vi "get_curr_position.vi"(8 "error in (no error)":errorcluster, 11 "XPS in":refnum<class "XPS.lvclass">) -> (0 "error out":errorcluster, 2 "readback position":dbl[](array[numeric]), 3 "XPS out":refnum<class "XPS.lvclass">)   [LabVIEW 2019, in "XPS.lvlib" / "XPS.lvclass"]
uses:
  XPS.lvclass
  XPS.lvclass/XPS.ctl
  Newport.XPS.CommandInterface
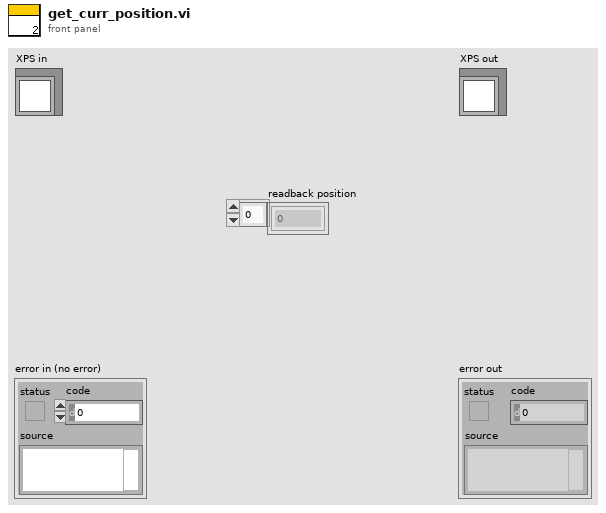
[diagram p1: front panel]
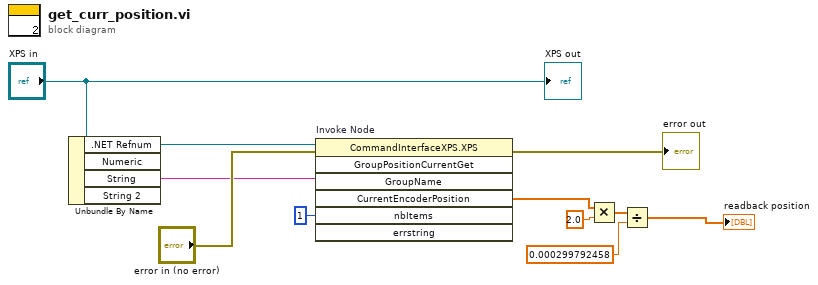
[diagram p0: block diagram]
diagram:
  n1 = Unbundle By Name("XPS in") -> (".NET Refnum"=w10:refnum<k24>, "String"=w1:string)  [unwired: 2 out]
  n2 = invoke on="Invoke Node" class="CommandInterfaceXPS.XPS" method="GroupPositionCurrentGet"(reference=w10, error in="error in (no error)", "GroupName"=w1, "nbItems"=1) -> (error out=→"error out":errorcluster, "CurrentEncoderPosition"=w4:dbl[])  [unwired: 3 in, 5 out]
  n3 = Multiply(x=w4, y=2.0) -> (x*y=w6:dbl[])
  n4 = Divide(x=w6, y=0.000299792458) -> (x/y=→"readback position":dbl[])
  "XPS out" <- "XPS in"
